vi "extract roi 2d.vi"(9 "ROI selected":i16, 10 "ROIs Array In":i32[][](array[numeric]), 11 "Data Form":T1) -> (2 "Table ROI 2D":i32[][](array[numeric]))   [LabVIEW 2023]
uses:
  control/Data Form.ctl
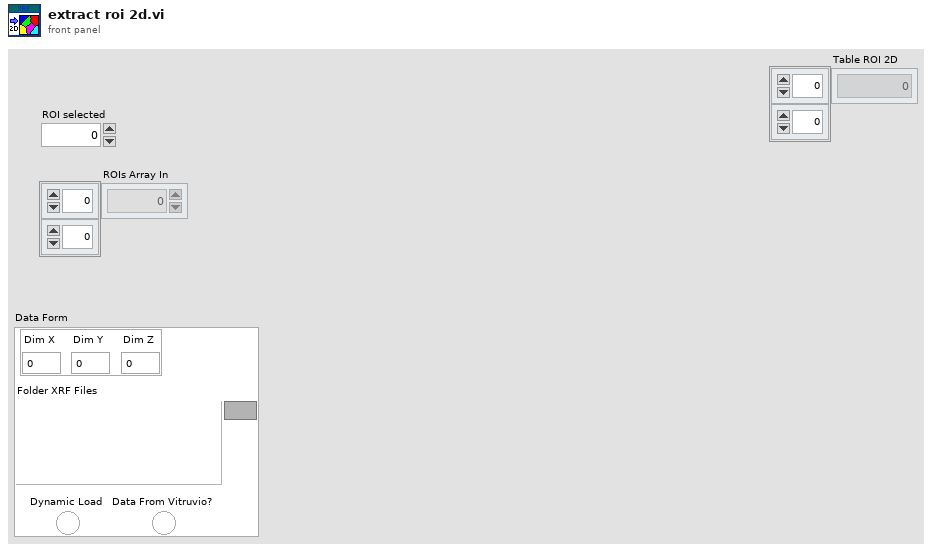
[diagram p1: front panel]
types:
  T1 = typedef "Data Form.ctl" = cluster{"Dimensions":cluster{"Dim X":i32, "Dim Y":i32, "Dim Z":i32}, "Folder XRF Files":path, "Dynamic Load":bool, "Data From Vitruvio?":bool}
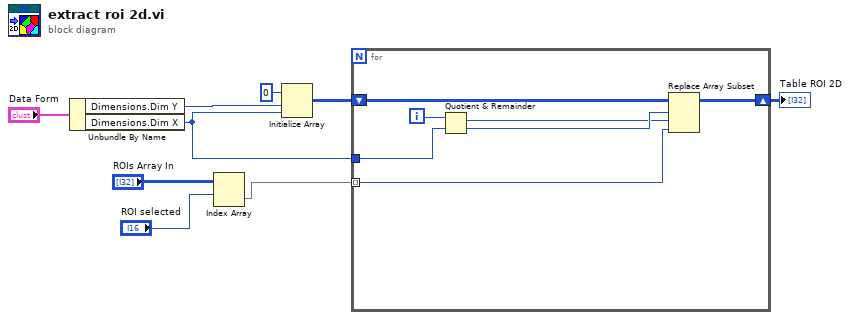
[diagram p0: block diagram]
diagram:
  n1 = Unbundle By Name("Data Form") -> ("Dimensions.Dim Y"=w7:i32, "Dimensions.Dim X"=w5:i32)
  n2 = Index Array(array="ROIs Array In", index (row)="ROI selected") -> (element=w2:i32[])  [unwired: 1 in]
  n3 = Initialize Array(0 ("element"), w7, w5) -> (w6:i32[][])
  n4 = for {
    tunnel: w2 -> [w10] mode=indexing
    shift-right: [w15] -> w4
    shift-left: w6 -> [w16]
    tunnel: w5 -> [w13]
    i -> [w14]
    n5 = Quotient & Remainder(x=w14, y=w13) -> (x-y*floor(x/y)=w11:i32, floor(x/y)=w12:i32)
    n6 = Replace Array Subset(array=w16, new element=w10, index (row)=w12, index (col)=w11) -> (w15:i32[][])
  }
  "Table ROI 2D" <- w4
